vi "Set App Config.vi"(8 "error in (no error)":errorcluster, 11 "Configuration":T1) -> (0 "error out":errorcluster)   [LabVIEW 2018]
uses:
  Controls/App Configuration.ctl
  <vilib>/Utility/xml.llb/Write to XML File(string).vi
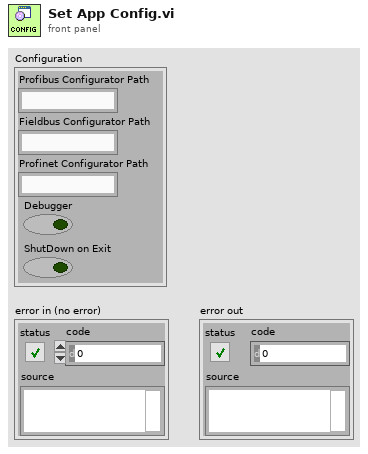
[diagram p1: front panel]
types:
  T1 = typedef "App Configuration.ctl" = cluster{"Profibus Configurator Path":string, "Fieldbus Configurator Path":string, "Profinet Configurator Path":string, "Debugger":bool, "ShutDown on Exit":bool}
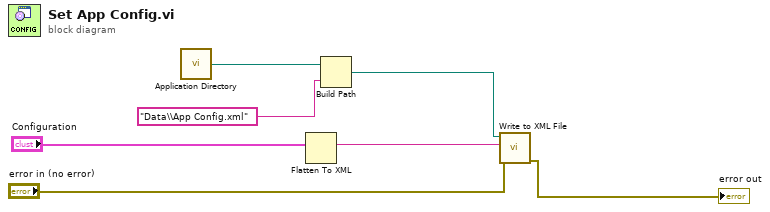
[diagram p0: block diagram]
diagram:
  n1 = call <vilib>:"Application Directory.vi"() -> ("Application Directory"=w2:path)
  n2 = Flatten To XML(anything="Configuration") -> (xml string=w5:string)
  n3 = Build Path(base path=w2, name or relative path="Data\\App Config.xml") -> (appended path=w1:path)
  n4 = call-poly <vilib>:"Write to XML File.vi"("error in (no error)"="error in (no error)", "XML Input"=w5, "XML File Path"=w1) -> ("error out"=→"error out":errorcluster)  [unwired: 6 in, 2 out]
